vi "gearSidePeg.vi"(11 "rightSide?":bool) -> ()   [LabVIEW 2016]
uses:
  <vilib>/Rock Robotics/WPI/Solenoid/WPI_SolenoidValue.ctl
  <vilib>/Rock Robotics/WPI/Solenoid/WPI_SolenoidSetEnum.vi
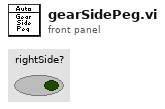
[diagram p1: front panel]
types:
  T1 = typedef "WPI_SolenoidValue.ctl" = enum16{"Off", "On", "Forward", "Reverse"}
  T2 = typedef "WPI_SolenoidDevRef.ctl" = cluster{"DevStatus":errorcluster, "Pneumatics Control Module":u8, "Forward Solenoid Channel":T3, "Reverse Solenoid Channel":T3}
  T3 = typedef "WPI_SolenoidChannel.ctl" = enum8{"Solenoid 0", "Solenoid 1", "Solenoid 2", "Solenoid 3", "Solenoid 4", "Solenoid 5", "Solenoid 6", "Solenoid 7", "Invalid"}
  T4 = typedef "WPI_MotorControlDeviceRef.ctl" = cluster{"DeviceStatus":errorcluster, "Type":T5, "PWM":cluster{"PWM Channel":T6, "DeadBand":T7}, "CAN":cluster{"Device Number":u8, "SetOutput VI Ref":variant, "GetOutput VI Ref":variant, "Enable VI Ref":variant, "Disable VI Ref":variant, "Data":variant}, "Invert":bool}
  T5 = typedef "WPI_MotorControlType.ctl" = enum16{"PWM", "CAN"}
  T6 = typedef "FPGA_DIOPWMChannel.ctl" = enum8{"PWM 0", "PWM 1", "PWM 2", "PWM 3", "PWM 4", "PWM 5", "PWM 6", "PWM 7", "PWM 8", "PWM 9", "PWM MXP 0", "PWM MXP 1", "PWM MXP 2", "PWM MXP 3", "PWM MXP 4", "PWM MXP 5", "PWM MXP 6", "PWM MXP 7", "PWM MXP 8", "PWM MXP 9", "Invalid"}
  T7 = typedef "WPI_PWMDeadband.ctl" = cluster{"Name":string, "maxPositivePwm":i32, "minPositivePwm":i32, "centerPwm":i32, "maxNegativePwm":i32, "minNegativePwm":i32, "angularRange":u16}
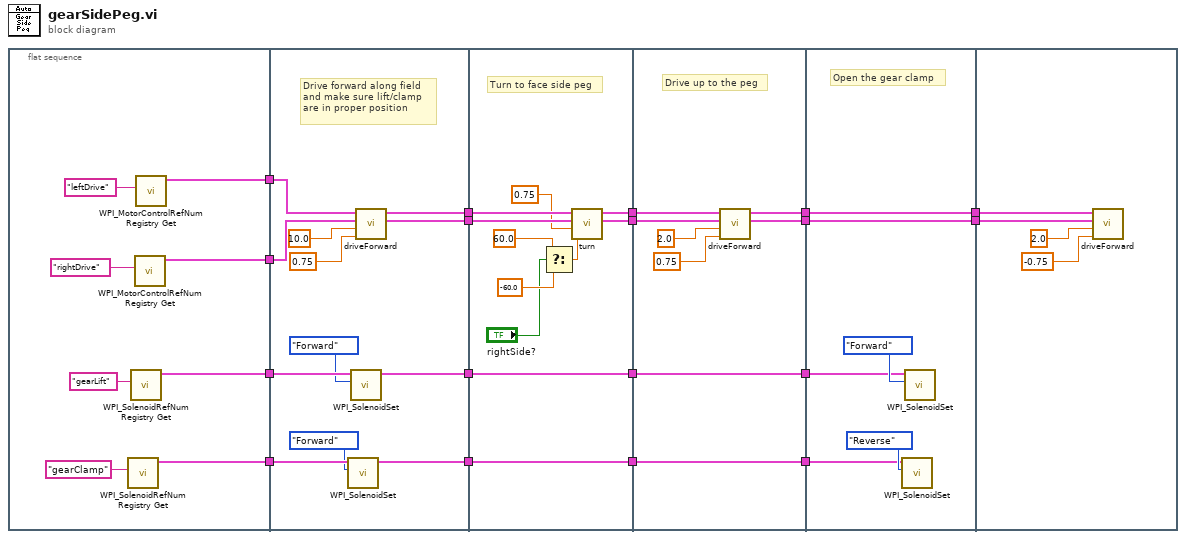
[diagram p0: block diagram]
diagram:
  n1 = flat-sequence {
    tunnel: [w22] -> w18
    tunnel: [w21] -> w17
    tunnel: [w20] -> w16
    tunnel: [w19] -> w15
    tunnel: w18 -> [w38]
    tunnel: w17 -> [w37]
    tunnel: w16 -> [w34]
    tunnel: w15 -> [w33]
    tunnel: [w30] -> w14
    tunnel: [w29] -> w13
    tunnel: [w28] -> w8
    tunnel: [w27] -> w5
    tunnel: w14 -> [w49]
    tunnel: w13 -> [w48]
    tunnel: [w42] -> w12
    tunnel: [w41] -> w11
    tunnel: [w40] -> w9
    tunnel: w8 -> [w40]
    tunnel: [w39] -> w6
    tunnel: w5 -> [w39]
    tunnel: w12 -> [w55]
    tunnel: w11 -> [w54]
    tunnel: [w53] -> w10
    tunnel: w9 -> [w53]
    tunnel: [w52] -> w7
    tunnel: w6 -> [w52]
    tunnel: [w51] -> w3
    tunnel: [w50] -> w2
    tunnel: w10 -> [w61]
    tunnel: w7 -> [w60]
    tunnel: [w59] -> w4
    tunnel: w3 -> [w59]
    tunnel: w2 -> [w58]
    tunnel: [w58] -> w1
    tunnel: w4 -> [w65]
    tunnel: w1 -> [w64]
    frame #0 {
      n2 = call <vilib>:"WPI_SolenoidRefNum Registry Get.vi"("refnum name"="gearClamp") -> ("SolenoidDevRef"=w19:T2)  [unwired: 9 in, 1 out]
      n3 = call <vilib>:"WPI_SolenoidRefNum Registry Get.vi"("refnum name"="gearLift") -> ("SolenoidDevRef"=w20:T2)  [unwired: 9 in, 1 out]
      n4 = call <vilib>:"WPI_MotorControlRefNum Registry Get.vi"("refnum name"="rightDrive") -> ("MotorControlDevRef"=w21:T4)  [unwired: 9 in, 1 out]
      n5 = call <vilib>:"WPI_MotorControlRefNum Registry Get.vi"("refnum name"="leftDrive") -> ("MotorControlDevRef"=w22:T4)  [unwired: 9 in, 1 out]
    }
    frame #1 {
      # "Drive forward along field\nand make sure lift/clamp\nare in proper position"
      n6 = call-poly <vilib>:"WPI_SolenoidSet.vi"("Value"=WPI_SolenoidValue."Forward", "SolenoidDevRef"=w33) -> ("SolenoidDevRef"=w27:T2)  [unwired: 8 in, 1 out]
      n7 = call-poly <vilib>:"WPI_SolenoidSet.vi"("Value"=WPI_SolenoidValue."Forward", "SolenoidDevRef"=w34) -> ("SolenoidDevRef"=w28:T2)  [unwired: 8 in, 1 out]
      n8 = call "driveForward.vi"("speed (%)"=0.75, "distance (ft)"=10.0, "rightMotor"=w37, "leftMotor"=w38) -> ("rightMotor"=w29:T4, "leftMotor"=w30:T4)  [unwired: 6 in]
    }
    frame #2 {
      # "Turn to face side peg"
      n9 = Select(t=60.0 ("angle (ccw)"), s="rightSide?", f=-60.0) -> (s? t:f=w45:dbl)
      n10 = call "turn.vi"("angle (ccw)"=w45, "speed (%)"=0.75, "rightMotor"=w48, "leftMotor"=w49) -> ("rightMotor"=w41:T4, "leftMotor"=w42:T4)  [unwired: 6 in]
    }
    frame #3 {
      # "Drive up to the peg"
      n11 = call "driveForward.vi"("speed (%)"=0.75, "distance (ft)"=2.0, "rightMotor"=w54, "leftMotor"=w55) -> ("rightMotor"=w50:T4, "leftMotor"=w51:T4)  [unwired: 6 in]
    }
    frame #4 {
      # "Open the gear clamp"
      n12 = call-poly <vilib>:"WPI_SolenoidSet.vi"("Value"=WPI_SolenoidValue."Reverse", "SolenoidDevRef"=w60) -> ()  [unwired: 8 in, 2 out]
      n13 = call-poly <vilib>:"WPI_SolenoidSet.vi"("Value"=WPI_SolenoidValue."Forward", "SolenoidDevRef"=w61) -> ()  [unwired: 8 in, 2 out]
    }
    frame #5 {
      n14 = call "driveForward.vi"("speed (%)"=-0.75, "distance (ft)"=2.0, "rightMotor"=w64, "leftMotor"=w65) -> ()  [unwired: 6 in, 2 out]
    }
  }
